vi "Control Examples.vi"() -> ()   [LabVIEW 2020]
uses:
  EquipmentVariant/Type Enum.ctl
  EquipmentVariant/EquipmentVariant.lvclass
  Robot/Robot.lvclass
  Pump/Pump.lvclass
panel:
  in  "EquipmentVariant":T1=enum."Instrument"
  in  "EquipmentVariant 3":cluster{"Instrument":refnum<visa-resource-name>}={"Instrument"="abc"}
  in  "EquipmentVariant":T1=enum."Instrument"
  in  "EquipmentVariant 2":cluster{"Pump":refnum<class "Pump.lvclass">}
  in  "EquipmentVariant":T2={"Robot"=refnum, "Pump"=refnum, "Instrument"="abc"}
  in  "EquipmentVariant":T1=enum."Instrument"
  in  "EquipmentVariant":cluster{"Robot":refnum<class "Robot.lvclass">}
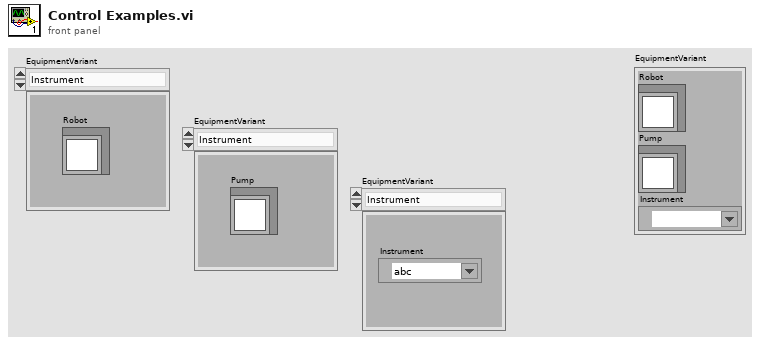
[diagram p1: front panel]
types:
  T1 = typedef "EquipmentVariant.lvclass/Type Enum.ctl" = enum16{"Robot", "Pump", "Instrument"}
  T2 = cluster{"Robot":refnum<class "Robot.lvclass">, "Pump":refnum<class "Pump.lvclass">, "Instrument":refnum<visa-resource-name>}
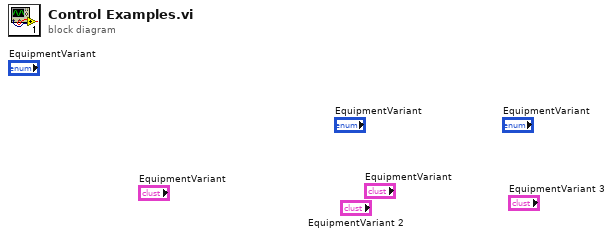
[diagram p0: block diagram]
diagram:
